vi "MIDI - Consumer.vi"(8 "error in (no error)":errorcluster, 11 "Queue in":refnum<queue>) -> (0 "error out":errorcluster, 3 "Queue out":refnum<queue>)   [LabVIEW 2014]
uses:
  MIDI/Controls/MidiCommand.ctl
  Controls/Application Data.vi
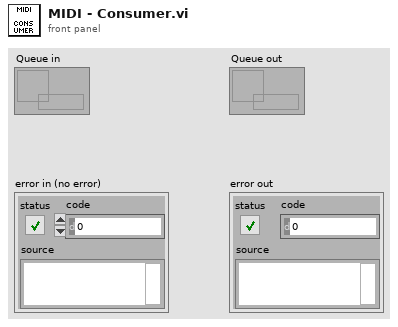
[diagram p1: front panel]
types:
  T1 = typedef "MidiCommand.ctl" = cluster{"Function":enum16{"Empty", "Note Off", "Note On", "Polyphonic Aftertouch", "Control/Mode Change", "Program Change", "Channel Aftertouch", "Pitch Bend Change", "System"}, "Channel":u8, "Data Byte 1":u8, "Data Byte 2":u8}
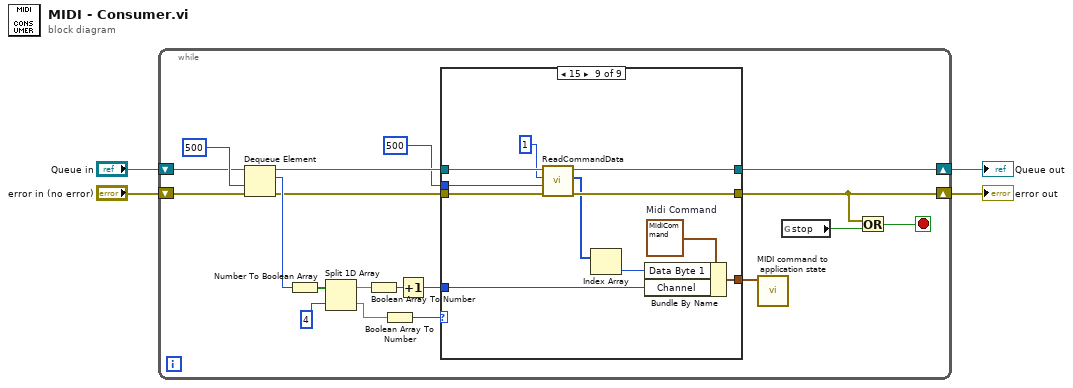
[diagram p0: block diagram]
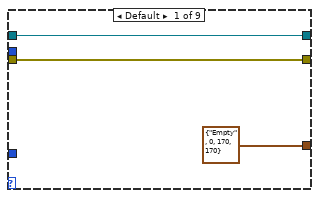
[diagram p2: hidden frame]
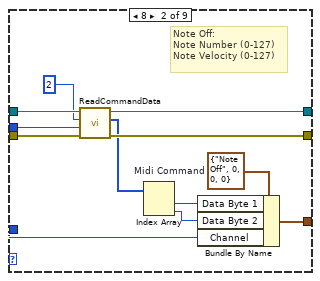
[diagram p3: hidden frame]
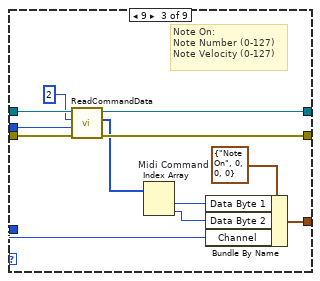
[diagram p4: hidden frame]
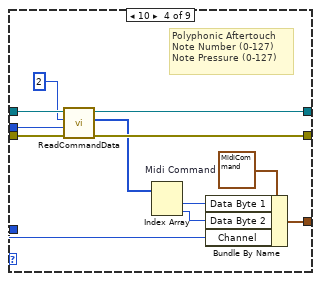
[diagram p5: hidden frame]
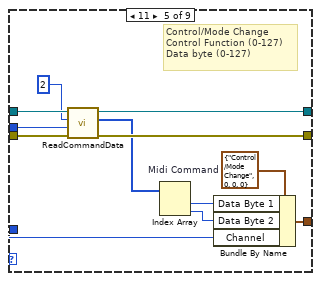
[diagram p6: hidden frame]
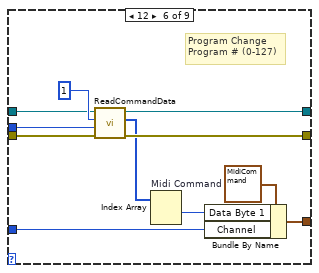
[diagram p7: hidden frame]
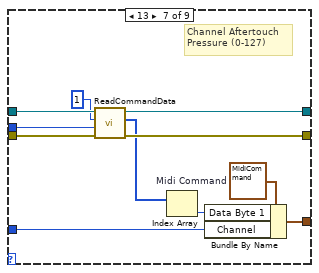
[diagram p8: hidden frame]
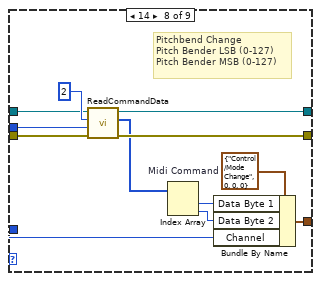
[diagram p9: hidden frame]
diagram:
  n1 = while {
    shift-right: [w7] -> w4
    shift-left: "error in (no error)" -> [w13]
    shift-right: [w21] -> w3
    shift-left: "Queue in" -> [w9]
    stop <- w8 stop-if-true
    n2 = Dequeue Element(queue=w9, timeout in ms (-1)=500, error in (no error)=w13) -> (queue out=w15:refnum<queue>, element=w20:u8, error out=w14:errorcluster)  [unwired: 1 out]
    n3 = Number To Boolean Array(number=w20) -> (Boolean array=w17:bool[])
    n4 = Split 1D Array(array=w17, index=4) -> (first subarray=w19:bool[], second subarray=w18:bool[])
    n5 = Boolean Array To Number(Boolean array=w19) -> (number=w5:u8)
    n6 = Boolean Array To Number(Boolean array=w18) -> (number=w11:u32)
    n7 = Increment(x=w5) -> (x+1=w16:u8)
    n8 = case shown="15" w11 {
      tunnel: [w25 w37 w47 w59 w72 w83 w94 w106 w118] -> w21
      tunnel: [w26 w29 w50 w61 w73 w84 w95 w107 w119] -> w7
      tunnel: w14 -> [w26 w38 w49 w62 w74 w85 w96 w108 w117]
      tunnel: w15 -> [w25 w36 w48 w60 w71 w81 w93 w104 w116]
      tunnel: 500 ("timeout in ms (-1)") -> [_ w34 w45 w57 w69 w80 w91 w103 w115]
      tunnel: [T1 {"Function"=enum."Empty", "Channel"=0, "Data Byte 1"=170, "Data Byte 2"=170} ("Midi Command") w32 w42 w55 w66 w78 w88 w100 w112] -> w23
      tunnel: w16 -> [_ w27 w39 w51 w64 w77 w86 w99 w110]
      frame Default {
      }
      frame 8 {
        w33 = T1 {"Function"=enum."Note Off", "Channel"=0, "Data Byte 1"=0, "Data Byte 2"=0}  # Midi Command
        # "Note Off: \nNote Number (0-127)\nNote Velocity (0-127)"
        n9 = call "ReadCommandData.vi"("error in (no error)"=w38, "timeout in ms (-1)"=w34, "Messages To Read"=u32 2, "Queue in"=w36) -> ("error out"=w29:errorcluster, "Data Bytes"=w28:u8[], "Queue in 2"=w37:refnum<queue>)  [unwired: 5 in]
        n10 = Index Array(array=w28) -> (element #1=w31:u8, element #2=w30:u8)  [unwired: 2 in]
        n11 = Bundle By Name(cluster=w33, "Data Byte 1"=w31, "Data Byte 2"=w30, "Channel"=w27) -> (w32:T1)
      }
      frame 9 {
        w43 = T1 {"Function"=enum."Note On", "Channel"=0, "Data Byte 1"=0, "Data Byte 2"=0}  # Midi Command
        # "Note On: \nNote Number (0-127)\nNote Velocity (0-127)"
        n12 = call "ReadCommandData.vi"("error in (no error)"=w49, "timeout in ms (-1)"=w45, "Messages To Read"=u32 2 ("byte count"), "Queue in"=w48) -> ("error out"=w50:errorcluster, "Data Bytes"=w40:u8[], "Queue in 2"=w47:refnum<queue>)  [unwired: 5 in]
        n13 = Index Array(array=w40) -> (element #1=w44:u8, element #2=w41:u8)  [unwired: 2 in]
        n14 = Bundle By Name(cluster=w43, "Data Byte 1"=w44, "Data Byte 2"=w41, "Channel"=w39) -> (w42:T1)
      }
      frame 10 {
        w56 = T1 {"Function"=enum."Polyphonic Aftertouch", "Channel"=0, "Data Byte 1"=0, "Data Byte 2"=0}  # Midi Command
        # "Polyphonic Aftertouch\nNote Number (0-127)\nNote Pressure (0-127)"
        n15 = call "ReadCommandData.vi"("error in (no error)"=w62, "timeout in ms (-1)"=w57, "Messages To Read"=u32 2 ("byte count"), "Queue in"=w60) -> ("error out"=w61:errorcluster, "Data Bytes"=w52:u8[], "Queue in 2"=w59:refnum<queue>)  [unwired: 5 in]
        n16 = Index Array(array=w52) -> (element #1=w54:u8, element #2=w53:u8)  [unwired: 2 in]
        n17 = Bundle By Name(cluster=w56, "Data Byte 1"=w54, "Data Byte 2"=w53, "Channel"=w51) -> (w55:T1)
      }
      frame 11 {
        w68 = T1 {"Function"=enum."Control/Mode Change", "Channel"=0, "Data Byte 1"=0, "Data Byte 2"=0}  # Midi Command
        # "Control/Mode Change\nControl Function (0-127)\nData byte (0-127)"
        n18 = call "ReadCommandData.vi"("error in (no error)"=w74, "timeout in ms (-1)"=w69, "Messages To Read"=u32 2 ("byte count"), "Queue in"=w71) -> ("error out"=w73:errorcluster, "Data Bytes"=w63:u8[], "Queue in 2"=w72:refnum<queue>)  [unwired: 5 in]
        n19 = Index Array(array=w63) -> (element #1=w67:u8, element #2=w65:u8)  [unwired: 2 in]
        n20 = Bundle By Name(cluster=w68, "Data Byte 1"=w67, "Data Byte 2"=w65, "Channel"=w64) -> (w66:T1)
      }
      frame 12 {
        w79 = T1 {"Function"=enum."Program Change", "Channel"=0, "Data Byte 1"=170, "Data Byte 2"=170}  # Midi Command
        # "Program Change\nProgram # (0-127)"
        n21 = call "ReadCommandData.vi"("error in (no error)"=w85, "timeout in ms (-1)"=w80, "Messages To Read"=u32 1 ("byte count"), "Queue in"=w81) -> ("error out"=w84:errorcluster, "Data Bytes"=w75:u8[], "Queue in 2"=w83:refnum<queue>)  [unwired: 5 in]
        n22 = Index Array(array=w75) -> (element #1=w76:u8)  [unwired: 2 in, 1 out]
        n23 = Bundle By Name(cluster=w79, "Data Byte 1"=w76, "Channel"=w77) -> (w78:T1)
      }
      frame 13 {
        w89 = T1 {"Function"=enum."Channel Aftertouch", "Channel"=0, "Data Byte 1"=170, "Data Byte 2"=170}  # Midi Command
        # "Channel Aftertouch\nPressure (0-127)"
        n24 = call "ReadCommandData.vi"("error in (no error)"=w96, "timeout in ms (-1)"=w91, "Messages To Read"=u32 1 ("byte count"), "Queue in"=w93) -> ("error out"=w95:errorcluster, "Data Bytes"=w87:u8[], "Queue in 2"=w94:refnum<queue>)  [unwired: 5 in]
        n25 = Index Array(array=w87) -> (element=w90:u8)  [unwired: 1 in]
        n26 = Bundle By Name(cluster=w89, "Data Byte 1"=w90, "Channel"=w86) -> (w88:T1)
      }
      frame 14 {
        w102 = T1 {"Function"=enum."Control/Mode Change", "Channel"=0, "Data Byte 1"=0, "Data Byte 2"=0}  # Midi Command
        # "Pitchbend Change\nPitch Bender LSB (0-127)\nPitch Bender MSB (0-127)"
        n27 = call "ReadCommandData.vi"("error in (no error)"=w108, "timeout in ms (-1)"=w103, "Messages To Read"=u32 2 ("byte count"), "Queue in"=w104) -> ("error out"=w107:errorcluster, "Data Bytes"=w97:u8[], "Queue in 2"=w106:refnum<queue>)  [unwired: 5 in]
        n28 = Index Array(array=w97) -> (element #1=w101:u8, element #2=w98:u8)  [unwired: 2 in]
        n29 = Bundle By Name(cluster=w102, "Data Byte 1"=w101, "Data Byte 2"=w98, "Channel"=w99) -> (w100:T1)
      }
      frame 15 {
        w114 = T1 {"Function"=enum."Program Change", "Channel"=0, "Data Byte 1"=170, "Data Byte 2"=170}  # Midi Command
        n30 = call "ReadCommandData.vi"("error in (no error)"=w117, "timeout in ms (-1)"=w115, "Messages To Read"=u32 1 ("byte count"), "Queue in"=w116) -> ("error out"=w119:errorcluster, "Data Bytes"=w111:u8[], "Queue in 2"=w118:refnum<queue>)  [unwired: 5 in]
        n31 = Index Array(array=w111) -> (element=w113:u8)  [unwired: 1 in]
        n32 = Bundle By Name(cluster=w114, "Data Byte 1"=w113, "Channel"=w110) -> (w112:T1)
      }
    }
    n33 = call "MIDI command to application state.vi"("Midi Command"=w23) -> ()  [unwired: 11 in]
    n34 = global read "Application Data.vi" "stop"() -> (w6:bool)
    n35 = Or(x=w7, y=w6) -> (x .or. y?=w8:bool)
  }
  "error out" <- w4
  "Queue out" <- w3
